vi "AD（V3.3）20M.vi"() -> ()   [LabVIEW 2013]
uses:
  ACTS1001_32.dll
panel:
  out "CH3 Data (mV)":sgl[](graph)
  out "CH2 Data (mV)":sgl[](graph)
  out "CH1 Data (mV)":sgl[](graph)
  out "CH0 Data (mV)":sgl[](graph)
  out "使能通道总数":i32
  out "要读取和处理的AD数据长度":u32
  in  "分频数":i32=20 min=1 step=1
  in  "是否为主设备":bool caption="触发输出使能"
  in  "时钟输出":i32(ring) items=["参考时钟", "基准时钟"]
  in  "时钟输出":bool caption="触发输出使能"
  in  "采样时基":i32(ring) items=["内部时钟", "外部时钟"]
  in  "参考时钟":i32(ring) items=["板载时钟", "外部10M", "PXI_CLK10M", "PXIe_CLK100M"]
  in  "输出宽度":i32=50 min=50 max=50000 step=50
  in  "触发输出使能":bool
  in  "触发输出":i32(ring) items=["负向触发", "正向触发", "正负向触发"]
  in  "延时点数":i32 min=0 step=1
  in  "停止":bool
  in  "同步信号触发源":i32(ring) items=["TRIG0信号", "TRIG1信号", "TRIG2信号", "TRIG3信号", "TRIG4信号", "TRIG5信号", "TRIG6信号", "TRIG7信号"]
  in  "触发电平":i32=1 min=1 max=10 step=1
  in  "触发灵敏窗":i32=1 min=1 max=255 step=1
  in  "触发方向":i32(ring) items=["下降沿触发", "上升沿触发", "上升沿下降沿均触发"]
  in  "触发模式":i32(ring) items=["后触发", "硬件延时触发"]
  in  "触发源":i32(ring) items=["软件触发", "外部数字触发", "同步信号触发", "通道0触发", "通道1触发", "通道2触发", "通道3触发"]
  out "采样频率":i32=10000 min=1 max=80000000 step=1
  in  "耦合类型1":i32(ring) items=["直流", "交流"]
  in  "CH0":bool=TRUE
  in  "耦合类型0":i32(ring) items=["直流", "交流"]
  in  "CH1":bool=TRUE
  in  "耦合类型2":i32(ring) items=["直流", "交流"]
  in  "CH2":bool=TRUE
  in  "耦合类型3":i32(ring) items=["直流", "交流"]
  in  "CH3":bool=TRUE
  in  "量程选择 0":i32(ring) items=["±5000mV"=0, "±1000mV"=2]
  in  "量程选择 1":i32(ring) items=["±5000mV"=0, "±1000mV"=2]
  in  "量程选择 2":i32(ring) items=["±5000mV"=0, "±1000mV"=2]
  in  "量程选择 3":i32(ring) items=["±5000mV"=0, "±1000mV"=2]
  # "各通道参数"
  # "通道选择"
  # "量程选择"
  # "耦合类型"
  # "支持使能方式：0通道；0和1通道；0、1、2和3通道"
  # "mV"
  # "nS"
  # "nS"
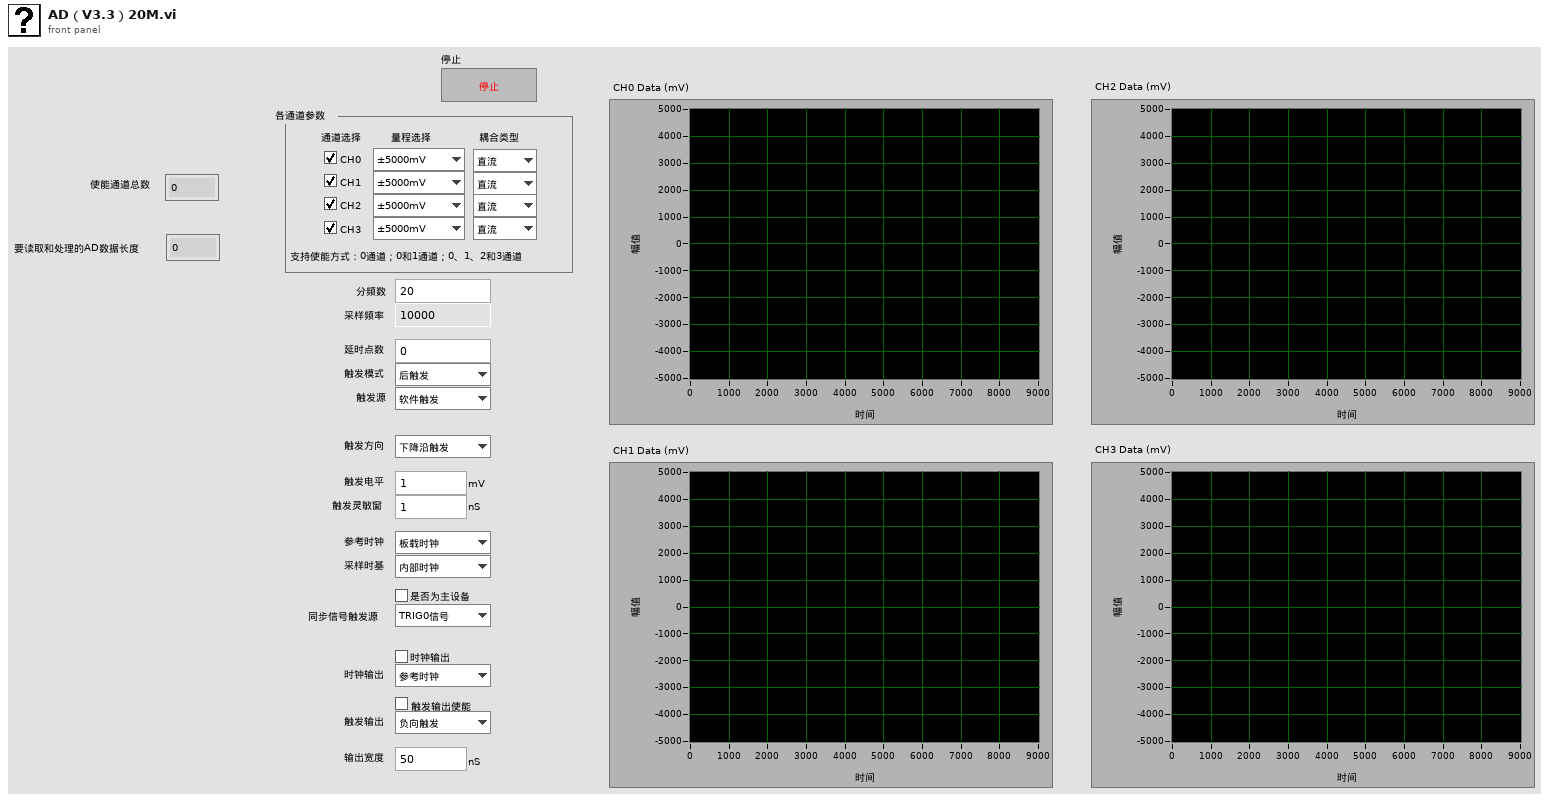
[diagram p1: front panel]
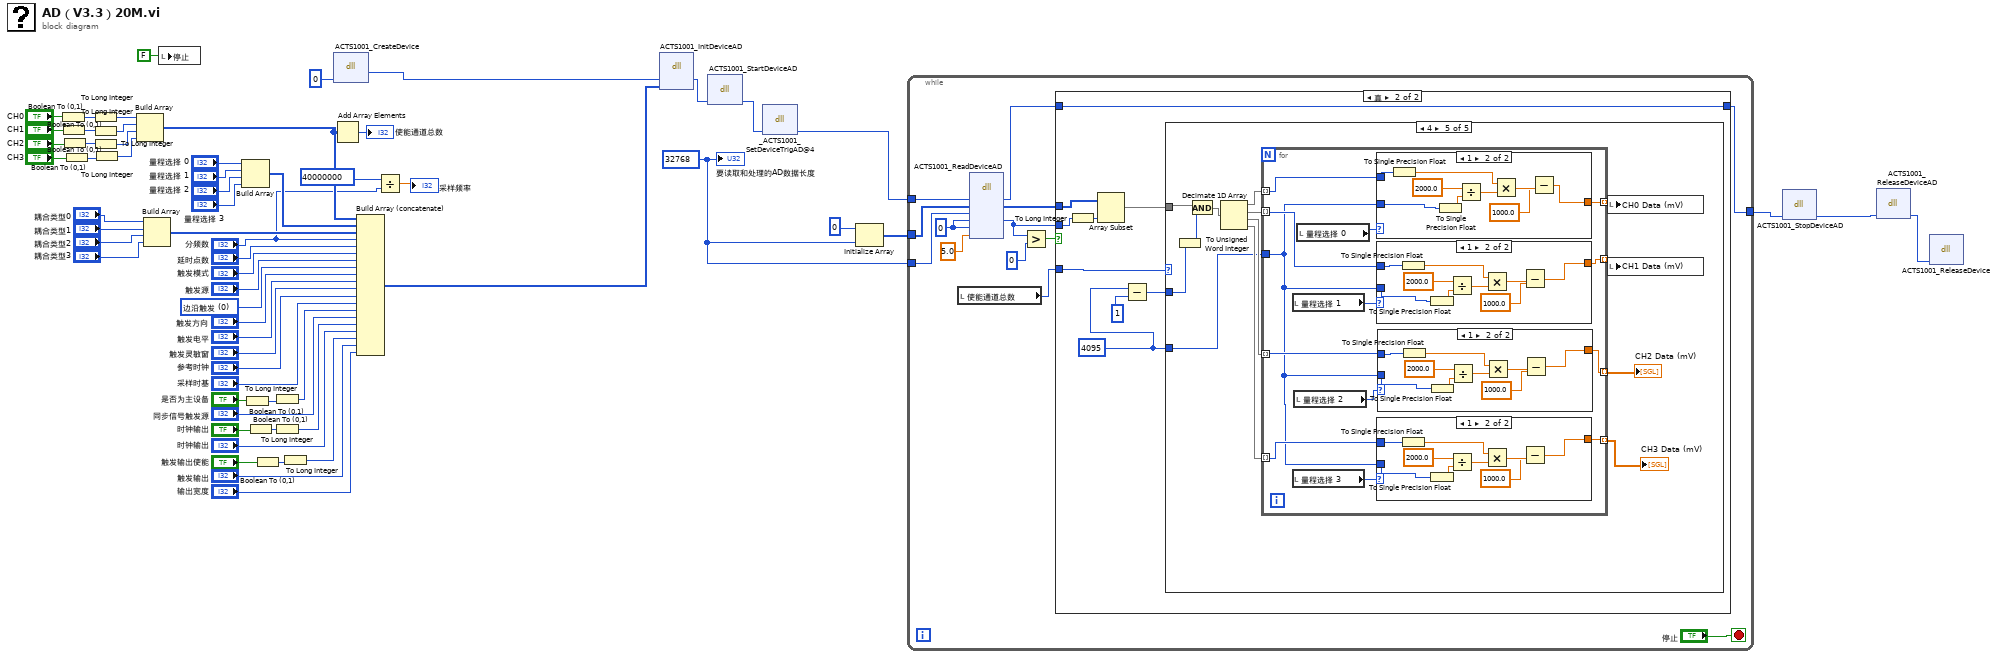
[diagram p0: block diagram]
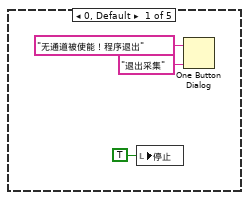
[diagram p3: hidden frame]
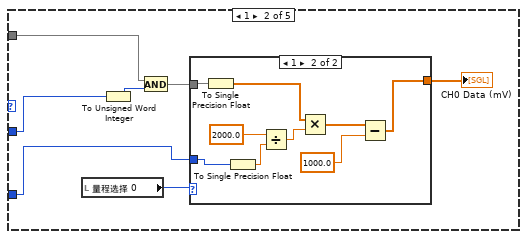
[diagram p4: hidden frame]
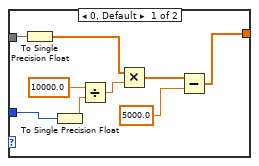
[diagram p5: hidden frame]
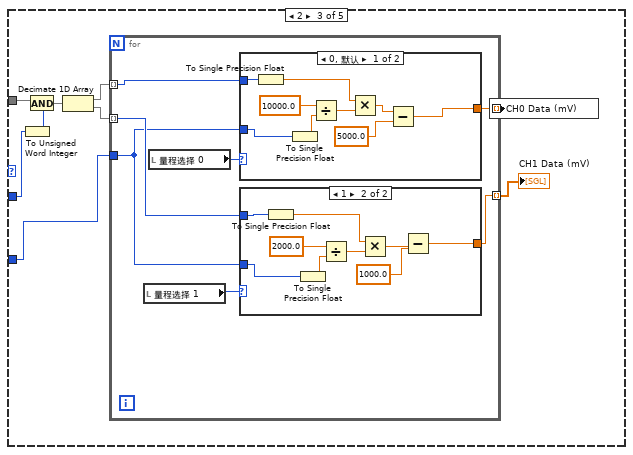
[diagram p6: hidden frame]
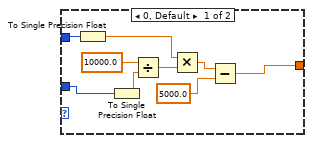
[diagram p7: hidden frame]
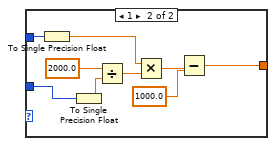
[diagram p8: hidden frame]
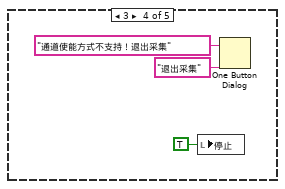
[diagram p9: hidden frame]
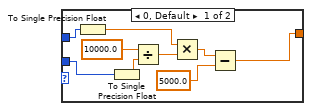
[diagram p10: hidden frame]
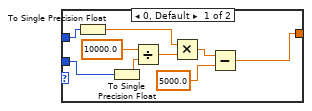
[diagram p11: hidden frame]
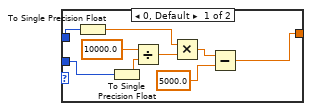
[diagram p12: hidden frame]
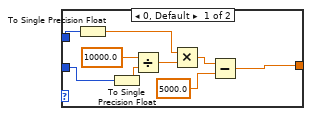
[diagram p13: hidden frame]
diagram:
  w28 = 0 items=["边沿触发", "脉冲触发"] ("触发类型")
  w7 = u32 32768 ("采样编码数量 2")
  n1 = Boolean To (0,1)(Boolean="CH0") -> (0, 1=w57:i16)
  n2 = Boolean To (0,1)(Boolean="CH1") -> (0, 1=w56:i16)
  n3 = Boolean To (0,1)(Boolean="CH2") -> (0, 1=w55:i16)
  n4 = Boolean To (0,1)(Boolean="CH3") -> (0, 1=w54:i16)
  n5 = To Long Integer(number=w57) -> (32bit integer=w46:i32)
  n6 = To Long Integer(number=w56) -> (32bit integer=w45:i32)
  n7 = To Long Integer(number=w55) -> (32bit integer=w44:i32)
  n8 = To Long Integer(number=w54) -> (32bit integer=w43:i32)
  n9 = Build Array(w46, w45, w44, w43) -> (w32:i32[])
  n10 = Build Array("耦合类型0", "耦合类型1", "耦合类型2", "耦合类型3") -> (w33:i32[])
  n11 = local write "停止"(FALSE ("停止")) -> ()
  n12 = Build Array("量程选择 0", "量程选择 1", "量程选择 2", "量程选择 3") -> (w38:i32[])
  n13 = Boolean To (0,1)(Boolean="是否为主设备") -> (0, 1=w22:i16)
  n14 = Boolean To (0,1)(Boolean="时钟输出") -> (0, 1=w21:i16)
  n15 = Boolean To (0,1)(Boolean="触发输出使能") -> (0, 1=w20:i16)
  n16 = To Long Integer(number=w22) -> (32bit integer=w18:i32)
  n17 = To Long Integer(number=w21) -> (32bit integer=w15:i32)
  n18 = To Long Integer(number=w20) -> (32bit integer=w13:i32)
  n19 = dll-call lib="ACTS1001_32.dll" fn="ACTS1001_CreateDevice"("DeviceLgcID"=0) -> ("hDevice"=w4:i32)  [unwired: 4 in, 2 out]
  n20 = Add Array Elements(numeric array=w32) -> (sum=→"使能通道总数":i32)
  n21 = Build Array (concatenate)(w32, w38, w33, "分频数", "延时点数", "触发模式", "触发源", w28, "触发方向", "触发电平", "触发灵敏窗", "参考时钟", "采样时基", w18, "同步信号触发源", w15, "时钟输出", w13, "触发输出", "输出宽度") -> (w53:i32[])
  n22 = Divide(x=40000000, y="分频数") -> (x/y=→"采样频率":dbl)
  n23 = dll-call lib="ACTS1001_32.dll" fn="ACTS1001_InitDeviceAD"("hDevice"=w4, "pADPara"=w53) -> ("hDevice"=w52:i32)  [unwired: 5 in, 2 out]
  n24 = dll-call lib="ACTS1001_32.dll" fn="ACTS1001_StartDeviceAD"("hDevice"=w52) -> ("hDevice"=w9:i32)  [unwired: 4 in, 2 out]
  n25 = dll-call lib="ACTS1001_32.dll" fn="_ACTS1001_SetDeviceTrigAD@4" label="ACTS1001_SetDeviceTrigAD"("hDevice"=w9) -> ("hDevice"=w8:i32)  [unwired: 4 in, 2 out]
  n26 = Initialize Array(u16 0, w7) -> (w48:u16[])
  n27 = while {
    tunnel: w8 -> [w75]
    tunnel: w48 -> [w74]
    tunnel: w7 -> [w72]
    tunnel: [w66] -> w6
    stop <- "停止" stop-if-true
    w71 = u32 0 ("RetReadSizeULongs")
    n28 = local read "使能通道总数"() -> (w63:i32)
    n29 = dll-call lib="ACTS1001_32.dll" fn="ACTS1001_ReadDeviceAD"("hDevice"=w75, "pADBuffer"=w74, "nReadSizeWords"=w72, "nRetSizeWords"=w71, "pAvailSampsPoints"=w71, "fTimeout"=5.0) -> ("hDevice"=w67:i32, "pADBuffer"=w65:u16[], "nRetSizeWords"=w64:u32)  [unwired: 7 in, 2 out]
    n30 = Greater?(x=w64, y=u32 0) -> (0:w68:bool)
    n31 = case shown="真" w68 {
      tunnel: w67 -> [w76 w85]
      tunnel: [w76 w85] -> w66
      tunnel: w65 -> [_ w82]
      tunnel: w64 -> [_ w80]
      tunnel: w63 -> [_ w84]
      frame False {
      }
      frame True {
        w77 = u16 4095
        n32 = To Long Integer(number=w80) -> (32bit integer=w83:i32)
        n33 = Array Subset(array=w82, length=w83) -> (w81:u16[])  [unwired: 1 in]
        n34 = Subtract(x=w77, y=1) -> (x-y=w78:i32)
        n35 = case shown="4" w84 {
          tunnel: w81 -> [_ w92 w119 _ w177]
          tunnel: w78 -> [_ w89 w114 _ w170]
          tunnel: w77 -> [_ w90 w115 _ w169]
          frame 0, Default {
            n36 = local write "停止"(TRUE ("停止")) -> ()
            n37 = One Button Dialog(message="无通道被使能！程序退出" ("消息"), button name ("OK")="退出采集" ("按钮名称（“确定”）")) -> ()  [unwired: 1 out]
          }
          frame 1 {
            n38 = local read "量程选择 0"() -> (w93:i32)
            n39 = To Unsigned Word Integer(number=w89) -> (unsigned 16bit integer=w94:u16)
            n40 = And(x=w92, y=w94) -> (x .and. y?=w95:u16[])
            n41 = case shown="1" w93 {
              tunnel: w95 -> [w104 w113]
              tunnel: [w99 w108] -> w91
              tunnel: w90 -> [w96 w105]
              frame 0, Default {
                n42 = To Single Precision Float(number=w104) -> (single precision float=w102:sgl[])
                n43 = To Single Precision Float(number=w96) -> (single precision float=w97:sgl)
                n44 = Divide(x=sgl 10000.0, y=w97) -> (x/y=w103:sgl)
                n45 = Multiply(x=w102, y=w103) -> (x*y=w101:sgl[])
                n46 = Subtract(x=w101, y=sgl 5000.0) -> (x-y=w99:sgl[])
              }
              frame 1 {
                n47 = To Single Precision Float(number=w113) -> (single precision float=w111:sgl[])
                n48 = To Single Precision Float(number=w105) -> (single precision float=w106:sgl)
                n49 = Divide(x=sgl 2000.0, y=w106) -> (x/y=w112:sgl)
                n50 = Multiply(x=w111, y=w112) -> (x*y=w110:sgl[])
                n51 = Subtract(x=w110, y=sgl 1000.0) -> (x-y=w108:sgl[])
              }
            }
            "CH0 Data (mV)" <- w91
          }
          frame 2 {
            n52 = To Unsigned Word Integer(number=w114) -> (unsigned 16bit integer=w120:u16)
            n53 = And(x=w119, y=w120) -> (x .and. y?=w118:u16[])
            n54 = Decimate 1D Array(w118) -> (w122:u16[], w121:u16[])
            n55 = for {
              tunnel: w122 -> [w128] mode=indexing
              tunnel: w121 -> [w126] mode=indexing
              tunnel: w115 -> [w125]
              tunnel: [w124] -> w117 mode=indexing
              tunnel: [w123] -> w116 mode=indexing
              n56 = local read "量程选择 1"() -> (w127:i32)
              n57 = local read "量程选择 0"() -> (w129:i32)
              n58 = case shown="0, 默认" w129 {
                tunnel: w128 -> [w156 w165]
                tunnel: [w151 w160] -> w124
                tunnel: w125 -> [w148 w157]
                frame 0, Default {
                  n59 = To Single Precision Float(number=w156) -> (single precision float=w154:sgl)
                  n60 = To Single Precision Float(number=w148) -> (single precision float=w149:sgl)
                  n61 = Divide(x=sgl 10000.0, y=w149) -> (x/y=w155:sgl)
                  n62 = Multiply(x=w154, y=w155) -> (x*y=w153:sgl)
                  n63 = Subtract(x=w153, y=sgl 5000.0) -> (x-y=w151:sgl)
                }
                frame 1 {
                  n64 = To Single Precision Float(number=w165) -> (single precision float=w163:sgl)
                  n65 = To Single Precision Float(number=w157) -> (single precision float=w158:sgl)
                  n66 = Divide(x=sgl 2000.0, y=w158) -> (x/y=w164:sgl)
                  n67 = Multiply(x=w163, y=w164) -> (x*y=w162:sgl)
                  n68 = Subtract(x=w162, y=sgl 1000.0) -> (x-y=w160:sgl)
                }
              }
              n69 = case shown="1" w127 {
                tunnel: w126 -> [w138 w147]
                tunnel: [w133 w142] -> w123
                tunnel: w125 -> [w130 w139]
                frame 0, Default {
                  n70 = To Single Precision Float(number=w138) -> (single precision float=w136:sgl)
                  n71 = To Single Precision Float(number=w130) -> (single precision float=w131:sgl)
                  n72 = Divide(x=sgl 10000.0, y=w131) -> (x/y=w137:sgl)
                  n73 = Multiply(x=w136, y=w137) -> (x*y=w135:sgl)
                  n74 = Subtract(x=w135, y=sgl 5000.0) -> (x-y=w133:sgl)
                }
                frame 1 {
                  n75 = To Single Precision Float(number=w147) -> (single precision float=w145:sgl)
                  n76 = To Single Precision Float(number=w139) -> (single precision float=w140:sgl)
                  n77 = Divide(x=sgl 2000.0, y=w140) -> (x/y=w146:sgl)
                  n78 = Multiply(x=w145, y=w146) -> (x*y=w144:sgl)
                  n79 = Subtract(x=w144, y=sgl 1000.0) -> (x-y=w142:sgl)
                }
              }
            }
            "CH1 Data (mV)" <- w116
            n80 = local write "CH0 Data (mV)"(w117) -> ()
          }
          frame 3 {
            n81 = local write "停止"(TRUE ("停止")) -> ()
            n82 = One Button Dialog(message="通道使能方式不支持！退出采集" ("消息"), button name ("OK")="退出采集" ("按钮名称（“确定”）")) -> ()  [unwired: 1 out]
          }
          frame 4 {
            n83 = To Unsigned Word Integer(number=w170) -> (unsigned 16bit integer=w179:u16)
            n84 = And(x=w177, y=w179) -> (x .and. y?=w178:u16[])
            n85 = Decimate 1D Array(w178) -> (w181:u16[], w180:u16[], w176:u16[], w175:u16[])
            n86 = for {
              tunnel: w181 -> [w193] mode=indexing
              tunnel: w180 -> [w191] mode=indexing
              tunnel: w169 -> [w182]
              tunnel: [w190] -> w172 mode=indexing
              tunnel: [w189] -> w171 mode=indexing
              tunnel: w176 -> [w188] mode=indexing
              tunnel: w175 -> [w187] mode=indexing
              tunnel: [w186] -> w174 mode=indexing
              tunnel: [w185] -> w173 mode=indexing
              n87 = local read "量程选择 1"() -> (w192:i32)
              n88 = local read "量程选择 3"() -> (w183:i32)
              n89 = local read "量程选择 2"() -> (w184:i32)
              n90 = local read "量程选择 0"() -> (w194:i32)
              n91 = case shown="1" w194 {
                tunnel: w193 -> [w257 w266]
                tunnel: [w252 w261] -> w190
                tunnel: w182 -> [w249 w258]
                frame 0, Default {
                  n92 = To Single Precision Float(number=w257) -> (single precision float=w255:sgl)
                  n93 = To Single Precision Float(number=w249) -> (single precision float=w250:sgl)
                  n94 = Divide(x=sgl 10000.0, y=w250) -> (x/y=w256:sgl)
                  n95 = Multiply(x=w255, y=w256) -> (x*y=w254:sgl)
                  n96 = Subtract(x=w254, y=sgl 5000.0) -> (x-y=w252:sgl)
                }
                frame 1 {
                  n97 = To Single Precision Float(number=w266) -> (single precision float=w264:sgl)
                  n98 = To Single Precision Float(number=w258) -> (single precision float=w259:sgl)
                  n99 = Divide(x=sgl 2000.0, y=w259) -> (x/y=w265:sgl)
                  n100 = Multiply(x=w264, y=w265) -> (x*y=w263:sgl)
                  n101 = Subtract(x=w263, y=sgl 1000.0) -> (x-y=w261:sgl)
                }
              }
              n102 = case shown="1" w192 {
                tunnel: w191 -> [w239 w248]
                tunnel: [w234 w243] -> w189
                tunnel: w182 -> [w231 w240]
                frame 0, Default {
                  n103 = To Single Precision Float(number=w239) -> (single precision float=w237:sgl)
                  n104 = To Single Precision Float(number=w231) -> (single precision float=w232:sgl)
                  n105 = Divide(x=sgl 10000.0, y=w232) -> (x/y=w238:sgl)
                  n106 = Multiply(x=w237, y=w238) -> (x*y=w236:sgl)
                  n107 = Subtract(x=w236, y=sgl 5000.0) -> (x-y=w234:sgl)
                }
                frame 1 {
                  n108 = To Single Precision Float(number=w248) -> (single precision float=w246:sgl)
                  n109 = To Single Precision Float(number=w240) -> (single precision float=w241:sgl)
                  n110 = Divide(x=sgl 2000.0, y=w241) -> (x/y=w247:sgl)
                  n111 = Multiply(x=w246, y=w247) -> (x*y=w245:sgl)
                  n112 = Subtract(x=w245, y=sgl 1000.0) -> (x-y=w243:sgl)
                }
              }
              n113 = case shown="1" w183 {
                tunnel: w187 -> [w203 w212]
                tunnel: [w198 w207] -> w186
                tunnel: w182 -> [w195 w204]
                frame 0, Default {
                  n114 = To Single Precision Float(number=w203) -> (single precision float=w201:sgl)
                  n115 = To Single Precision Float(number=w195) -> (single precision float=w196:sgl)
                  n116 = Divide(x=sgl 10000.0, y=w196) -> (x/y=w202:sgl)
                  n117 = Multiply(x=w201, y=w202) -> (x*y=w200:sgl)
                  n118 = Subtract(x=w200, y=sgl 5000.0) -> (x-y=w198:sgl)
                }
                frame 1 {
                  n119 = To Single Precision Float(number=w212) -> (single precision float=w210:sgl)
                  n120 = To Single Precision Float(number=w204) -> (single precision float=w205:sgl)
                  n121 = Divide(x=sgl 2000.0, y=w205) -> (x/y=w211:sgl)
                  n122 = Multiply(x=w210, y=w211) -> (x*y=w209:sgl)
                  n123 = Subtract(x=w209, y=sgl 1000.0) -> (x-y=w207:sgl)
                }
              }
              n124 = case shown="1" w184 {
                tunnel: w188 -> [w214 w230]
                tunnel: [w217 w225] -> w185
                tunnel: w182 -> [w213 w222]
                frame 0, Default {
                  n125 = To Single Precision Float(number=w214) -> (single precision float=w220:sgl)
                  n126 = To Single Precision Float(number=w213) -> (single precision float=w215:sgl)
                  n127 = Divide(x=sgl 10000.0, y=w215) -> (x/y=w221:sgl)
                  n128 = Multiply(x=w220, y=w221) -> (x*y=w219:sgl)
                  n129 = Subtract(x=w219, y=sgl 5000.0) -> (x-y=w217:sgl)
                }
                frame 1 {
                  n130 = To Single Precision Float(number=w230) -> (single precision float=w228:sgl)
                  n131 = To Single Precision Float(number=w222) -> (single precision float=w223:sgl)
                  n132 = Divide(x=sgl 2000.0, y=w223) -> (x/y=w229:sgl)
                  n133 = Multiply(x=w228, y=w229) -> (x*y=w227:sgl)
                  n134 = Subtract(x=w227, y=sgl 1000.0) -> (x-y=w225:sgl)
                }
              }
            }
            "CH2 Data (mV)" <- w173
            "CH3 Data (mV)" <- w174
            n135 = local write "CH0 Data (mV)"(w172) -> ()
            n136 = local write "CH1 Data (mV)"(w171) -> ()
          }
        }
      }
    }
  }
  n137 = dll-call lib="ACTS1001_32.dll" fn="ACTS1001_StopDeviceAD" label="StopDeviceAD"("hDevice"=w6) -> ("hDevice"=w51:i32)  [unwired: 4 in, 2 out]
  n138 = dll-call lib="ACTS1001_32.dll" fn="ACTS1001_ReleaseDeviceAD" label="ReleaseDeviceAD"("hDevice"=w51) -> ("hDevice"=w50:i32)  [unwired: 4 in, 2 out]
  n139 = dll-call lib="ACTS1001_32.dll" fn="ACTS1001_ReleaseDevice" label="ReleaseDevice"("hDevice"=w50) -> ()  [unwired: 5 in, 2 out]
  "要读取和处理的AD数据长度" <- w7
